vi "PresentStatus.vi"() -> ()   [LabVIEW 2012]
panel:
  in  "演示模式":enum16{"在线检测", "离线回放"}(ring)
  in  "当前状态":enum16{"等待状态", "重新开始", "正常工作", "退出系统"}(ring)
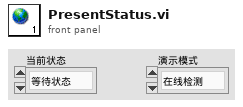
[diagram p1: front panel]
diagram:
